vi "Read InitOptions.vi"(8 "error in (no error)":errorcluster, 11 "ScopePluginsBase in":refnum<class "ScopePluginsBase.lvclass">) -> (0 "error out":errorcluster, 2 "InitOptions":T1, 3 "ScopePluginsBase out":refnum<class "ScopePluginsBase.lvclass">)   [LabVIEW 2018, in "ScopePlugins.lvlib" / "ScopePluginsBase.lvclass"]
uses:
  ScopePluginsBase.lvclass
  TypeDefs/InitializeOptions.ctl
  ScopePluginsBase.lvclass/ScopePluginsBase.ctl
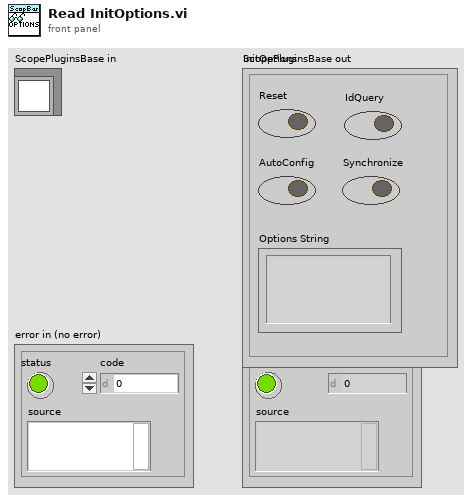
[diagram p1: front panel]
types:
  T1 = typedef "ScopePlugins.lvlib/ScopePluginsBase.lvclass/InitializeOptions.ctl" = cluster{"Reset":bool, "IdQuery":bool, "AutoConfig":bool, "Options String":string, "Synchronize":bool}
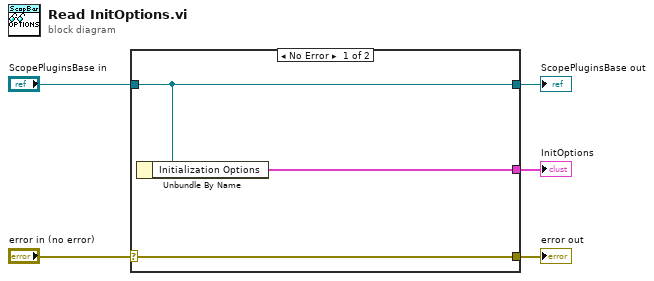
[diagram p0: block diagram]
diagram:
  n1 = case shown="No Error" "error in (no error)" {
    selector: "error in (no error)" -> [w8 w9]
    tunnel: [w8 w9] -> w4
    tunnel: [w7 w10] -> w2
    tunnel: "ScopePluginsBase in" -> [w7 w10]
    tunnel: [w6 _] -> w1
    frame No Error {
      n2 = Unbundle By Name(w7) -> ("Initialization Options"=w6:T1)
    }
    frame Error {
    }
  }
  "error out" <- w4
  "ScopePluginsBase out" <- w2
  "InitOptions" <- w1
